vi "device class selection.vi"(3 "detect all (F)":bool, 6 "custom device class":string[](array[string]), 7 "device classes":T1) -> (1 "device class":string[](array[string]))   [LabVIEW 2016, in "SMI.lvlib" / "Device.lvclass"]
uses:
  Device.lvclass
  device class selection.ctl
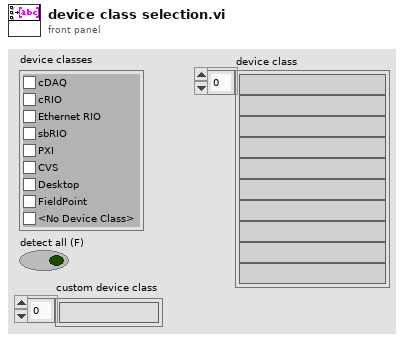
[diagram p1: front panel]
types:
  T1 = typedef "SMI.lvlib/Device.lvclass/device class selection.ctl" = cluster{"cDAQ":bool, "cRIO":bool, "Ethernet RIO":bool, "sbRIO":bool, "PXI":bool, "CVS":bool, "Desktop":bool, "FieldPoint":bool, "<No Device Class>":bool}
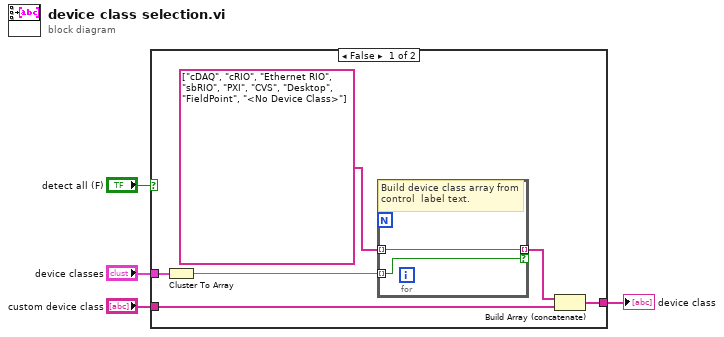
[diagram p0: block diagram]
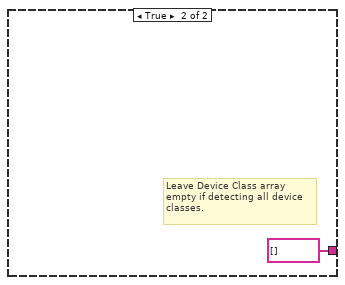
[diagram p2: hidden frame]
diagram:
  n1 = case shown="False" "detect all (F)" {
    tunnel: "device classes" -> [w10 _]
    tunnel: "custom device class" -> [w7 _]
    tunnel: [w6 string[] []] -> w2
    frame False {
      n2 = Cluster To Array(cluster=w10) -> (array=w9:bool[])
      n3 = for {
        tunnel: w9 -> [w12] mode=indexing
        tunnel: [w11] -> w8 mode=indexing if=w12
        tunnel: string[] ["cDAQ", "cRIO", "Ethernet RIO", "sbRIO", "PXI", "CVS", "Desktop", "FieldPoint", "<No Device Class>"] -> [w11] mode=indexing
        # "Build device class array from control  label text."
      }
      n4 = Build Array (concatenate)(w8, w7) -> (w6:string[])
    }
    frame True {
      # "Leave Device Class array\nempty if detecting all device\nclasses."
    }
  }
  "device class" <- w2
